vi "readTestDescription.vi"(8 "error in (no error)":errorcluster, 11 "Prueba02 in":refnum<class "Prueba02.lvclass">) -> (0 "error out":errorcluster, 2 "Test Description":string, 3 "Prueba02 out":refnum<class "Prueba02.lvclass">)   [LabVIEW 2019, in "Prueba02.lvclass"]
uses:
  Prueba02.lvclass
  Prueba02.lvclass/Prueba02.ctl
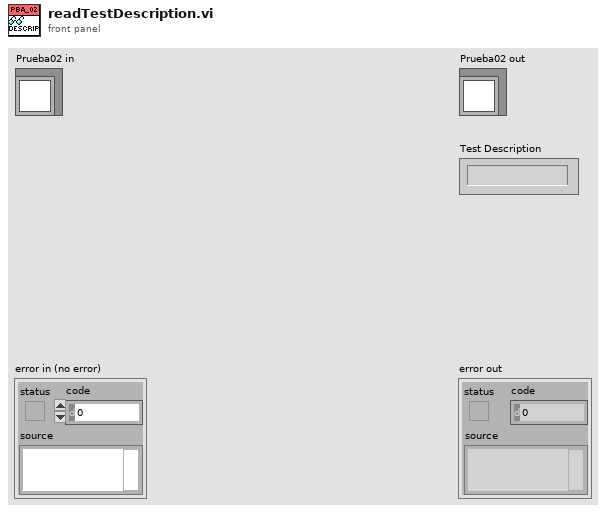
[diagram p1: front panel]
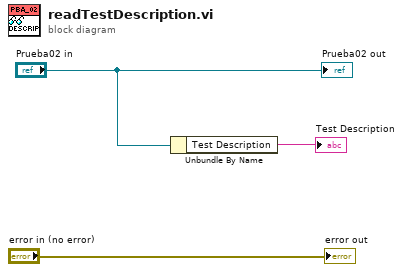
[diagram p0: block diagram]
diagram:
  n1 = Unbundle By Name("Prueba02 in") -> ("Test Description"=→"Test Description":string)
  "error out" <- "error in (no error)"
  "Prueba02 out" <- "Prueba02 in"
